vi "Item Sibling Index.vi"(0 "Tree Reference In":refnum<vi>, 2 "Child Tag (Current)":string, 5 "error in (no error)":errorcluster) -> (14 "Tree Reference Out":refnum<vi>, 15 "Parent Tag":string, 16 "Child Tag Dub":string, 17 "Index Among Siblings":i32, 19 "error out":errorcluster)   [LabVIEW 2015, in "QuickVIew.lvlib"]
doc: "Retrieves the top down index of an element amongst its siblings.\n\nex. If a parent has 4 children A,B,C,D in that respective top down order this function would return 2 for a child tag input of CTLB Prime - Application Template 1.3.0.24\nNorm Kirchner, NI Systems Engineering - NI\nCopyright (c) 2014, NI"
uses:
  QuickVIew.lvlib
panel:
  # "VI INPUTS"
  # "VI OUTPUTS"
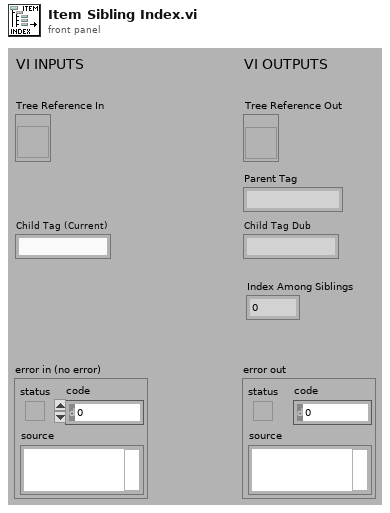
[diagram p1: front panel]
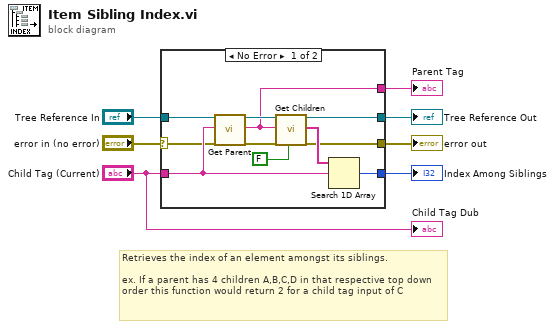
[diagram p0: block diagram]
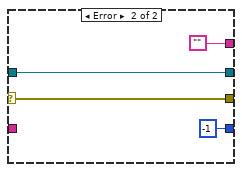
[diagram p2: hidden frame]
diagram:
  # "Retrieves the index of an element amongst its siblings.\n\nex. If a parent has 4 children A,B,C,D in that respective top down order this function would return 2 for a child tag input of C"
  n1 = case shown="No Error" "error in (no error)" {
    selector: "error in (no error)" -> [w11 w21]
    tunnel: "Child Tag (Current)" -> [w15 _]
    tunnel: "Tree Reference In" -> [w13 w22]
    tunnel: [w12 w21] -> w6
    tunnel: [w10 -1 ("index of element")] -> w4
    tunnel: [w9 w22] -> w3
    tunnel: [w8 ""] -> w1
    frame No Error {
      n2 = call "Get Parent.vi"("Tree Reference In"=w13, "Child Tag (Current)"=w15, "error in (no error)"=w11) -> ("Tree Reference Out"=w18:refnum<vi>, "Parent Tag"=w8:string, "error out"=w17:errorcluster)  [unwired: 13 in, 1 out]
      n3 = call "Get Children.vi"("Tree Reference In"=w18, "Parent Tag"=w8, "error in (no error)"=w17, "Use Current"=FALSE) -> ("Tree Reference Out"=w9:refnum<vi>, "Children Tags"=w16:string[], "error out"=w12:errorcluster)  [unwired: 13 in]
      n4 = Search 1D Array(1D array=w16, element=w15) -> (index of element=w10:i32)  [unwired: 1 in]
    }
    frame Error {
    }
  }
  "error out" <- w6
  "Index Among Siblings" <- w4
  "Tree Reference Out" <- w3
  "Parent Tag" <- w1
  "Child Tag Dub" <- "Child Tag (Current)"
